vi "co2Read.vi"() -> ()   [LabVIEW 2019]
uses:
  <vilib>/Instr/_visa.llb/VISA Configure Serial Port (Instr).vi
panel:
  out "t6":dbl
  out "h6":dbl caption="h4"
  out "zone 3":dbl
  out "t5":dbl
  out "t4":dbl
  out "t3":dbl
  out "t2":dbl
  out "h5":dbl
  out "h4":dbl
  out "h3":dbl
  out "h2":dbl
  out "zone 1":dbl
  out "outlet":dbl
  out "zone 2":dbl
  out "main return":dbl
  out "h1":dbl
  out "t1":dbl
  out "inlet air":dbl
  in  "VISA- Arduino Uno":refnum<visa-resource-name>
  in  "stop":bool
  # "CO2\n\n\n\nTemperature\n\n\n\nHumidity"
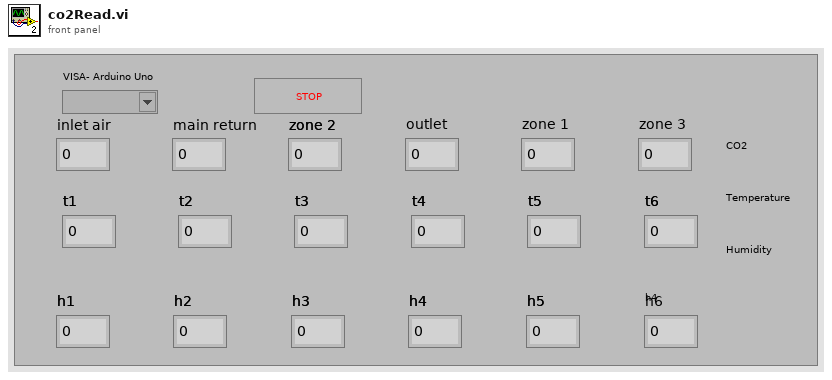
[diagram p1: front panel]
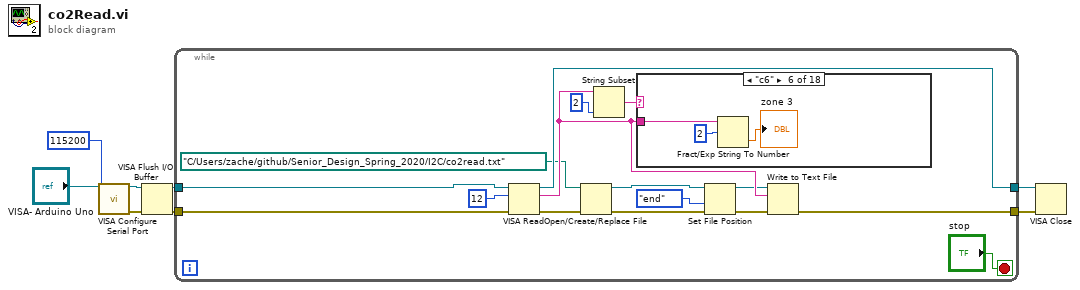
[diagram p0: block diagram]
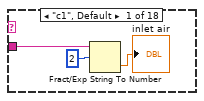
[diagram p2: hidden frame]
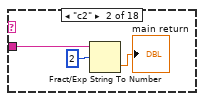
[diagram p3: hidden frame]
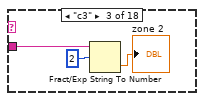
[diagram p4: hidden frame]
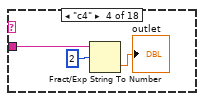
[diagram p5: hidden frame]
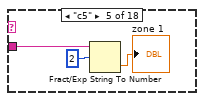
[diagram p6: hidden frame]
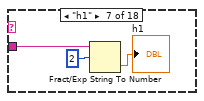
[diagram p7: hidden frame]
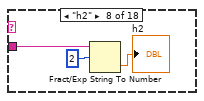
[diagram p8: hidden frame]
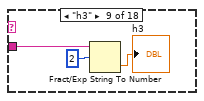
[diagram p9: hidden frame]
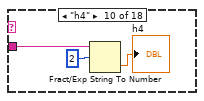
[diagram p10: hidden frame]
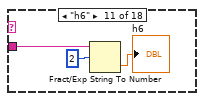
[diagram p11: hidden frame]
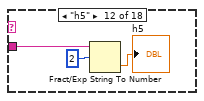
[diagram p12: hidden frame]
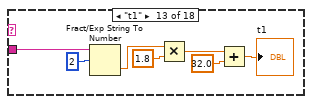
[diagram p13: hidden frame]
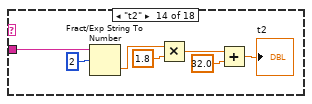
[diagram p14: hidden frame]
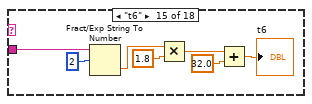
[diagram p15: hidden frame]
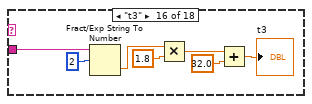
[diagram p16: hidden frame]
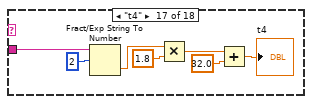
[diagram p17: hidden frame]
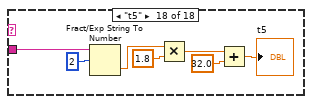
[diagram p18: hidden frame]
diagram:
  n1 = call-poly "VISA Configure Serial Port"("VISA resource name"="VISA- Arduino Uno", "baud rate (115200)"=u32 115200) -> ("VISA resource name out"=w5:refnum<visa-resource-name>, "error out"=w6:errorcluster)  [unwired: 12 in]
  n2 = VISA Flush I/O Buffer(VISA resource name=w5, error in (no error)=w6) -> (VISA resource name out=w7:refnum<visa-resource-name>, error out=w4:errorcluster)  [unwired: 1 in]
  n3 = while {
    tunnel: w7 -> [w21]
    tunnel: w4 -> [w22]
    tunnel: [w18] -> w3
    tunnel: [w16] -> w2
    stop <- "stop" stop-if-true
    n4 = VISA Read(VISA resource name=w21, byte count=u32 12, error in (no error)=w22) -> (VISA resource name out=w18:refnum<visa-resource-name>, read buffer=w17:string, error out=w12:errorcluster)  [unwired: 1 out]
    n5 = Open/Create/Replace File(file path (use dialog)=path "C:/Users/zache/github/Senior_Design_Spring_2020/I2C/co2read.txt" ("file (use dialog)"), error in=w12) -> (refnum out=w14:refnum<file>, error out=w15:errorcluster)  [unwired: 4 in, 1 out]
    n6 = String Subset(string=w17, length (rest)=2 ("length (rest)")) -> (substring=w20:string)  [unwired: 1 in]
    n7 = case shown="\"c6\"" w20 {
      tunnel: w17 -> [w26 w29 w32 w35 w38 w41 w44 w47 w50 w53 w56 w59 w66 w73 w80 w87 w94 w101]
      frame "c1", Default {
        n8 = Fract/Exp String To Number(string=w26, offset=2) -> (number=→"inlet air":dbl)  [unwired: 2 in, 1 out]
      }
      frame "c2" {
        n9 = Fract/Exp String To Number(string=w29, offset=2) -> (number=→"main return":dbl)  [unwired: 2 in, 1 out]
      }
      frame "c3" {
        n10 = Fract/Exp String To Number(string=w32, offset=2) -> (number=→"zone 2":dbl)  [unwired: 2 in, 1 out]
      }
      frame "c4" {
        n11 = Fract/Exp String To Number(string=w35, offset=2) -> (number=→"outlet":dbl)  [unwired: 2 in, 1 out]
      }
      frame "c5" {
        n12 = Fract/Exp String To Number(string=w38, offset=2) -> (number=→"zone 1":dbl)  [unwired: 2 in, 1 out]
      }
      frame "c6" {
        n13 = Fract/Exp String To Number(string=w41, offset=2) -> (number=→"zone 3":dbl)  [unwired: 2 in, 1 out]
      }
      frame "h1" {
        n14 = Fract/Exp String To Number(string=w44, offset=2) -> (number=→"h1":dbl)  [unwired: 2 in, 1 out]
      }
      frame "h2" {
        n15 = Fract/Exp String To Number(string=w47, offset=2) -> (number=→"h2":dbl)  [unwired: 2 in, 1 out]
      }
      frame "h3" {
        n16 = Fract/Exp String To Number(string=w50, offset=2) -> (number=→"h3":dbl)  [unwired: 2 in, 1 out]
      }
      frame "h4" {
        n17 = Fract/Exp String To Number(string=w53, offset=2) -> (number=→"h4":dbl)  [unwired: 2 in, 1 out]
      }
      frame "h6" {
        n18 = Fract/Exp String To Number(string=w56, offset=2) -> (number=→"h6":dbl)  [unwired: 2 in, 1 out]
      }
      frame "h5" {
        n19 = Fract/Exp String To Number(string=w59, offset=2) -> (number=→"h5":dbl)  [unwired: 2 in, 1 out]
      }
      frame "t1" {
        n20 = Fract/Exp String To Number(string=w66, offset=2) -> (number=w62:dbl)  [unwired: 2 in, 1 out]
        n21 = Multiply(x=w62, y=1.8) -> (x*y=w64:dbl)
        n22 = Add(x=w64, y=32.0) -> (x+y=→"t1":dbl)
      }
      frame "t2" {
        n23 = Fract/Exp String To Number(string=w73, offset=2) -> (number=w69:dbl)  [unwired: 2 in, 1 out]
        n24 = Multiply(x=w69, y=1.8) -> (x*y=w71:dbl)
        n25 = Add(x=w71, y=32.0) -> (x+y=→"t2":dbl)
      }
      frame "t6" {
        n26 = Fract/Exp String To Number(string=w80, offset=2) -> (number=w76:dbl)  [unwired: 2 in, 1 out]
        n27 = Multiply(x=w76, y=1.8) -> (x*y=w78:dbl)
        n28 = Add(x=w78, y=32.0) -> (x+y=→"t6":dbl)
      }
      frame "t3" {
        n29 = Fract/Exp String To Number(string=w87, offset=2) -> (number=w83:dbl)  [unwired: 2 in, 1 out]
        n30 = Multiply(x=w83, y=1.8) -> (x*y=w85:dbl)
        n31 = Add(x=w85, y=32.0) -> (x+y=→"t3":dbl)
      }
      frame "t4" {
        n32 = Fract/Exp String To Number(string=w94, offset=2) -> (number=w90:dbl)  [unwired: 2 in, 1 out]
        n33 = Multiply(x=w90, y=1.8) -> (x*y=w92:dbl)
        n34 = Add(x=w92, y=32.0) -> (x+y=→"t4":dbl)
      }
      frame "t5" {
        n35 = Fract/Exp String To Number(string=w101, offset=2) -> (number=w97:dbl)  [unwired: 2 in, 1 out]
        n36 = Multiply(x=w97, y=1.8) -> (x*y=w99:dbl)
        n37 = Add(x=w99, y=32.0) -> (x+y=→"t5":dbl)
      }
    }
    n38 = Set File Position(refnum=w14, from (0:start)=enum16{"start", "end", "current"}."end", error in=w15) -> (refnum out=w9:refnum<file>, error out=w11:errorcluster)  [unwired: 1 in]
    n39 = Write to Text File(file (use dialog)=w9, text=w17, error in=w11) -> (error out=w16:errorcluster)  [unwired: 1 in, 2 out]
  }
  n40 = VISA Close(VISA resource name=w3, error in (no error)=w2) -> ()  [unwired: 1 out]
